vi "TimerForTeacher.vi"(8 "error in (no error)":errorcluster, 11 "Time to Elapse (2s)":dbl=2.0) -> (0 "error out":errorcluster, 2 "Time Elapsed?":bool, 3 "Time Elapsed":dbl)   [LabVIEW 2020]
uses:
  #typedef_TimerAction.ctl
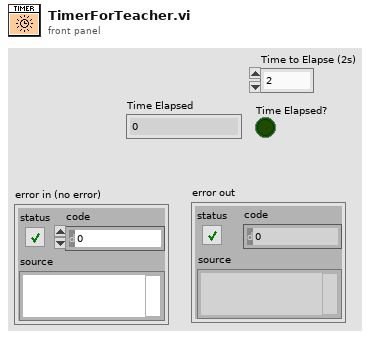
[diagram p1: front panel]
types:
  T1 = typedef "#typedef_TimerAction.ctl" = enum16{"Reset", "Time Elapsed"}
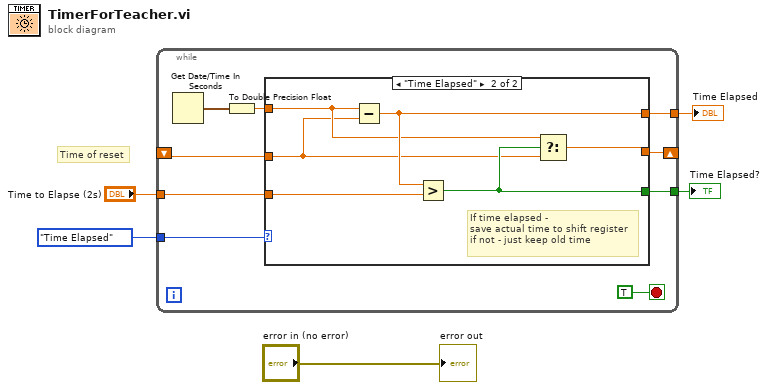
[diagram p0: block diagram]
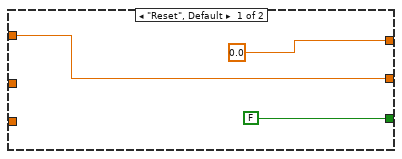
[diagram p2: hidden frame]
diagram:
  # "Time of reset"
  n1 = while {
    shift-right: [w10] -> _
    shift-left: _ -> [w11]
    tunnel: #typedef_TimerAction."Time Elapsed" ("Enum") -> [w14]
    tunnel: [w8] -> w5
    tunnel: [w7] -> w3
    tunnel: "Time to Elapse (2s)" -> [w6]
    stop <- TRUE stop-if-true
    n2 = Get Date/Time In Seconds() -> (seconds since 1Jan1904=w12:timestamp)
    n3 = To Double Precision Float(number=w12) -> (double precision float=w9:dbl)
    n4 = case shown="\"Time Elapsed\"" w14 {
      tunnel: w11 -> [_ w18]
      tunnel: [w17 w20] -> w10
      tunnel: w9 -> [w17 w19]
      tunnel: [0.0 w23] -> w8
      tunnel: [FALSE w21] -> w7
      tunnel: w6 -> [_ w22]
      frame "Reset", Default {
      }
      frame "Time Elapsed" {
        # "If time elapsed - \nsave actual time to shift register\nif not - just keep old time"
        n5 = Subtract(x=w19, y=w18) -> (x-y=w23:dbl)
        n6 = Greater?(x=w23, y=w22) -> (0:w21:bool)
        n7 = Select(t=w19, s=w21, f=w18) -> (s? t:f=w20:dbl)
      }
    }
  }
  "Time Elapsed" <- w5
  "Time Elapsed?" <- w3
  "error out" <- "error in (no error)"
